vi "ReadAll.vi"() -> ()   [LabVIEW 2015]
uses:
  <vilib>/rvi/interface/nirviMethod/nirviMethod.xnode
  <vilib>/rvi/interface/nirviReadWriteControl/nirviReadWriteControl.xnode
  <vilib>/Analysis/NI_AALPro.lvlib
  <vilib>/measure/NI_MAPro.lvlib
  <vilib>/measure/matone.llb/Extract Single Tone Information 1 Chan.vi
  <vilib>/rvi/interface/nirviOpenFPGA/nirviOpenFPGA.xnode
  <vilib>/rvi/interface/nirviCloseFPGA/nirviCloseFPGA.xnode
  FPGA Bitfiles/DloopFunds_FPGATarget_DunkFlips_5YK2PK4xqNI.lvbitx
  DunkFlips.vi
  <vilib>/FPGAPlugInAG/Dynamic/niLvFpga_ReadFifo_Dynamic.vi
  <vilib>/rvi/errors/niLvFpgaMergeErrorWithErrorCode.vi
  <vilib>/FPGAPlugInAG/Dynamic/niLvFpga_Close_Dynamic.vi
  <vilib>/FPGAPlugInAG/USB-7855R OEM/niLvFpga_Open_USB-7855R OEM.vi
  <vilib>/rvi/interface/common/dynamic/niFpgaDynamicAddResources.vi
  NiFpgaLv.dll
  <vilib>/Utility/error.llb/Error Cluster From Error Code.vi
  <vilib>/rvi/interface/Simulation/niFpgaSimulationCallBeginRW.vi
  <vilib>/rvi/errors/niLvFpgaAdjustHostInterfaceError.vi
panel:
  out "Output 3":i16
  out "Output 2":i16
  out "Output 1":i16
  in  "Requested Sample Period (ticks)":i16
  in  "Min signal time gap (samples)":i16
  in  "FIFO Signal":i16
  in  "Max Period (samples)":fxp<+/-,64,32>
  in  "Min Period (samples)":fxp<+/-,64,32>
  in  "Min Amplitude 4":fxp<+/-,64,32>
  in  "Min Amplitude 3":fxp<+/-,64,32>
  in  "Min Amplitude 2":fxp<+/-,64,32>
  in  "Min Amplitude 1":fxp<+/-,64,32>
  in  "High Pass":bool
  out "Signal":waveform(dbl)(graph)
  in  "Peak height":fxp<+/-,16,4>
  out "Output time":dbl
  in  "Low Pass":bool
  out "Frequ":dbl
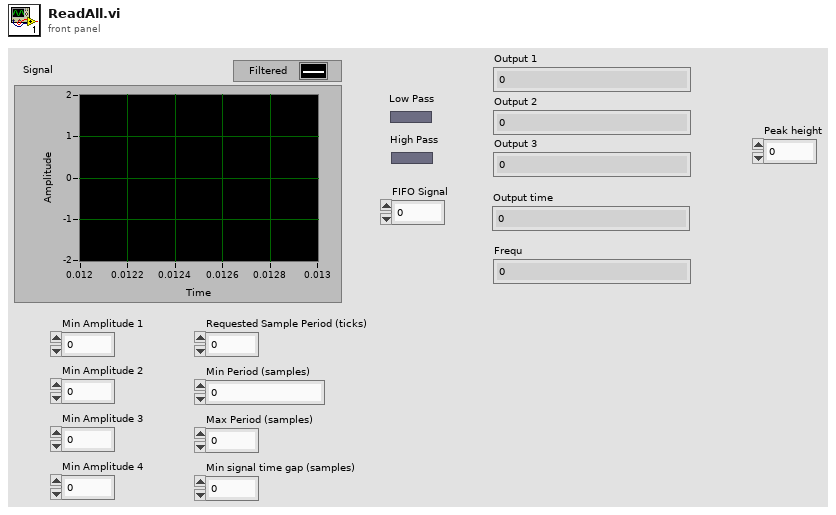
[diagram p1: front panel]
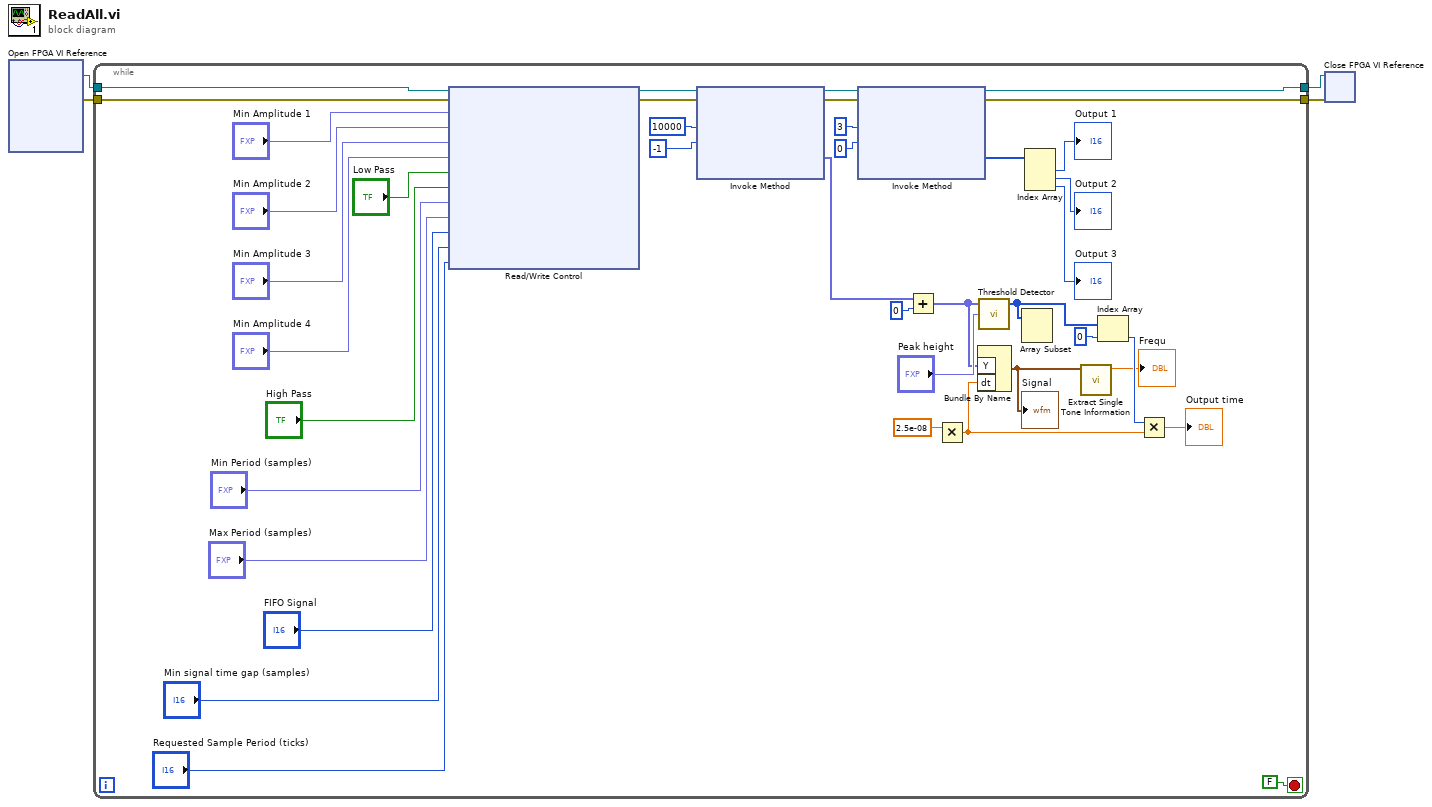
[diagram p0: block diagram]
diagram:
  n1 = xnode "Open FPGA VI Reference"() -> ("FPGA VI Reference Out"=w2:refnum<k20>, "error out"=w1:errorcluster)  [unwired: 2 in]
  n2 = while {
    tunnel: [w12] -> w4
    tunnel: [w11] -> w3
    tunnel: w2 -> [w42]
    tunnel: w1 -> [w41]
    stop <- FALSE stop-if-true
    n3 = xnode "Read/Write Control"("FPGA VI Reference In"=w42, "error in"=w41, "Min Amplitude 1"="Min Amplitude 1", "Min Amplitude 2"="Min Amplitude 2", "Min Amplitude 3"="Min Amplitude 3", "Min Amplitude 4"="Min Amplitude 4", "Low Pass"="Low Pass", "High Pass"="High Pass", "Min Period (samples)"="Min Period (samples)", "Max Period (samples)"="Max Period (samples)", "FIFO Signal"="FIFO Signal", "Min signal time gap (samples)"="Min signal time gap (samples)", "Requested Sample Period (ticks)"="Requested Sample Period (ticks)") -> ("FPGA VI Reference Out"=w39:refnum<k20>, "error out"=w40:errorcluster)
    n4 = xnode "Invoke Method"("FPGA VI Reference In"=w39, "error in"=w40, "Number of Elements"=10000, "Timeout (ms)"=-1) -> ("FPGA VI Reference Out"=w14:refnum<k20>, "error out"=w13:errorcluster, "Data"=w32:fxp<+/-,24,16>[])  [unwired: 1 out]
    n5 = xnode "Invoke Method"("FPGA VI Reference In"=w14, "error in"=w13, "Number of Elements"=3, "Timeout (ms)"=0) -> ("FPGA VI Reference Out"=w12:refnum<k20>, "error out"=w11:errorcluster, "Data"=w8:i32[])  [unwired: 1 out]
    n6 = Add(x=w32, y=0) -> (x+y=w31:fxp<+/-,41,33>[])
    n7 = Multiply(x=2.5e-08) -> (x*y=w34:dbl)  [unwired: 1 in]
    n8 = Bundle By Name("Y"=w31, "dt"=w34) -> (w17:waveform(dbl))  [unwired: 1 in]
    "Signal" <- w17
    n9 = call <vilib>:"Threshold Detector.vi"("threshold"="Peak height", "X"=w31) -> ("Indices"=w29:i32[])  [unwired: 1 in, 2 out]
    n10 = Array Subset(array=w29) -> ()  [unwired: 2 in, 1 out]
    n11 = Index Array(array=w8) -> (element #1=→"Output 1":i32, element #2=→"Output 2":i32, element #3=→"Output 3":i32)  [unwired: 3 in]
    n12 = call-poly <vilib>:"Extract Single Tone Information.vi"("time signal in"=w17) -> ("detected frequency"=→"Frequ":dbl)  [unwired: 5 in, 5 out]
    n13 = Index Array(array=w29, index=0) -> (element=w35:i32)
    n14 = Multiply(x=w35, y=w34) -> (x*y=→"Output time":dbl)
  }
  n15 = xnode "Close FPGA VI Reference"("FPGA VI Reference In"=w4, "error in"=w3) -> ()  [unwired: 1 out]
